vi "Get PWM Configuration.vi"(8 "error in":errorcluster, 10 "channels":refnum<class "Channel.lvclass">[](array[class]), 11 "mode in":refnum<class "Mode.lvclass">) -> (0 "error out":errorcluster, 2 "PWM":T1 {"PWM Channels"."PWM frequency" items=["1 Hz", "50 Hz", "250 Hz", "500 Hz", "1 kHz", "5 kHz", "10 kHz", "20 kHz"]}, 3 "mode out":refnum<class "Mode.lvclass">)   [LabVIEW 2017, in "Scan Engine Scripting.lvlib" / "Mode.lvclass"]
uses:
  Mode.lvclass
  Channel Classes/Channel/Channel.lvclass
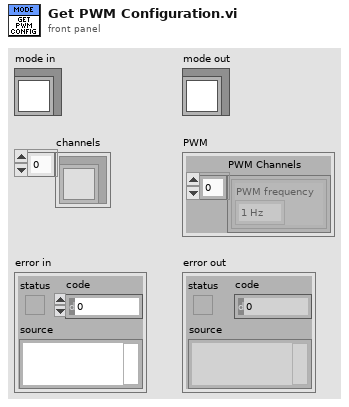
[diagram p1: front panel]
types:
  T1 = cluster{"PWM Channels":cluster{"PWM frequency":u32}[]}
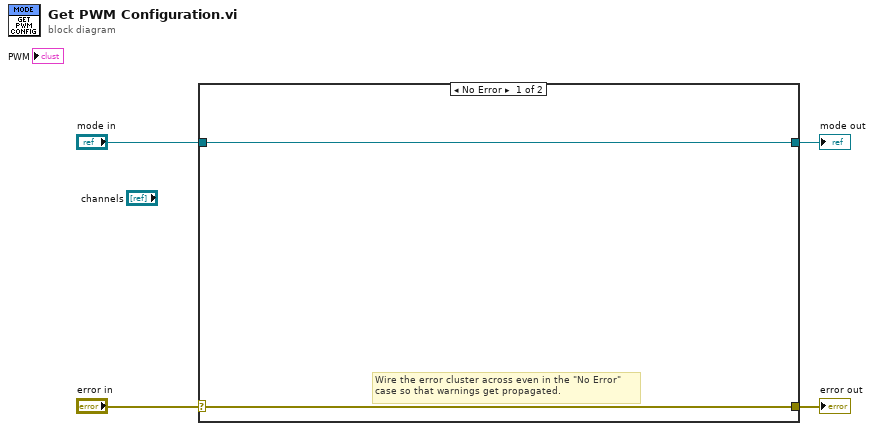
[diagram p0: block diagram]
diagram:
  n1 = case shown="No Error" "error in" {
    selector: "error in" -> [w5 w8]
    tunnel: [w5 w8] -> w3
    tunnel: [w6 w7] -> w1
    tunnel: "mode in" -> [w6 w7]
    frame No Error {
      # "Wire the error cluster across even in the \"No Error\"\ncase so that warnings get propagated."
    }
    frame Error {
    }
  }
  "error out" <- w3
  "mode out" <- w1
